vi "DoHandshake.vi"(6 "Additional Return headers (none)":T1[](array[typedef]), 8 "error in (no error)":errorcluster, 9 "timeout ms (5000)":i32=5000, 10 "Supported Protocols (any)":string[](array[string]), 11 "WebSocket Connection in":refnum<k5>) -> (0 "error out":errorcluster, 1 "Request URI":string, 2 "Headers Out":variant, 3 "WebSocket Connection out":refnum<k5>)   [LabVIEW 2013, in "WebSockets.lvlib"]
doc: "Performs the WebSockets HTTP handshaking on the new TCP connection. The client sends HTTP headers and the server must reply with a correctly formed HTTP response. The VI handles an incoming WS-Protocol and will return it in the response headers if it matches the supported protocols input. Additional HTTP headers can also be returned."
uses:
  WebSockets.lvlib
  Headers.ctl
panel:
  out "HTTP Headers":string
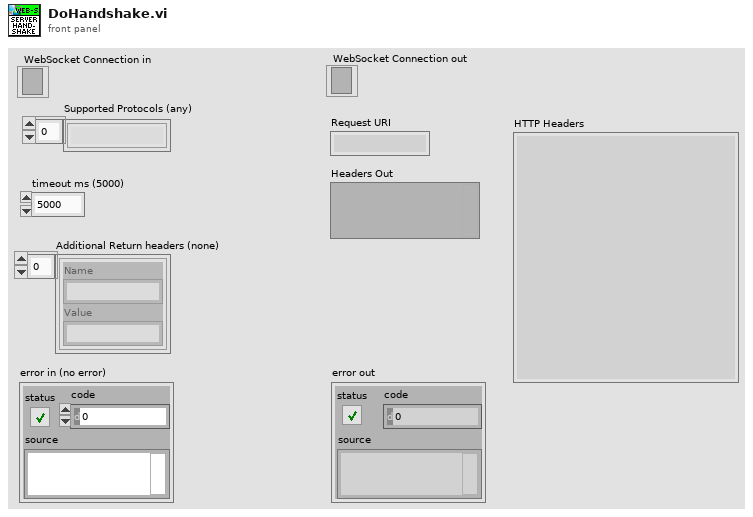
[diagram p1: front panel]
types:
  T1 = typedef "WebSockets.lvlib/Headers.ctl" = cluster{"Name":string, "Value":string}
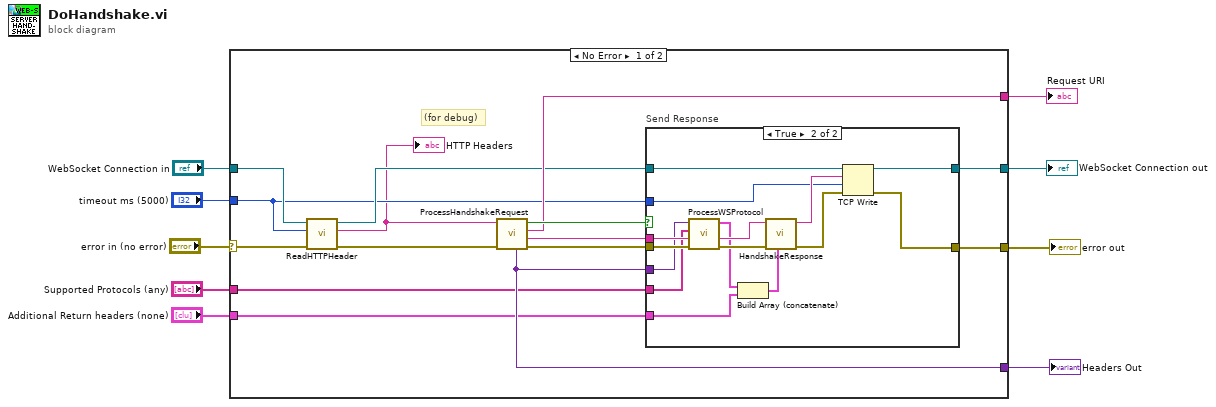
[diagram p0: block diagram]
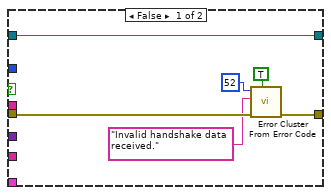
[diagram p2: hidden frame]
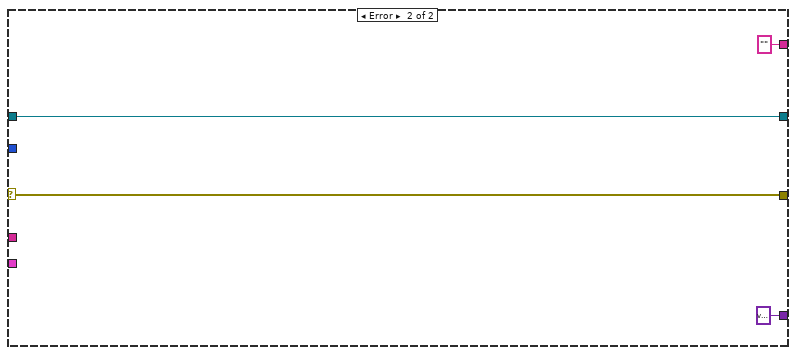
[diagram p3: hidden frame]
diagram:
  n1 = case shown="No Error" "error in (no error)" {
    selector: "error in (no error)" -> [w17 w48]
    tunnel: [w24 w47] -> w9
    tunnel: "WebSocket Connection in" -> [w18 w47]
    tunnel: [w20 w48] -> w6
    tunnel: "timeout ms (5000)" -> [w14 _]
    tunnel: [w12 variant ("Headers Out")] -> w4
    tunnel: [w19 "" ("Path")] -> w3
    tunnel: "Supported Protocols (any)" -> [w11 _]
    tunnel: "Additional Return headers (none)" -> [w10 _]
    frame No Error {
      # "(for debug)"
      n2 = call "ReadHTTPHeader.vi"("error in (no error)"=w17, "timeout ms (25000)"=w14, "WebSocket Connection in"=w18) -> ("error out"=w16:errorcluster, "HTTP Header"=w13:string, "WebSocket Connection out"=w15:refnum<k5>)  [unwired: 6 in]
      "HTTP Headers" <- w13
      n3 = call "ProcessHandshakeRequest.vi"("error in (no error)"=w16, "HTTP Headers"=w13) -> ("error out"=w21:errorcluster, "Sec-WebSocket-Key"=w23:string, "Path"=w19:string, "Is Websocket Request?"=w22:bool, "Headers Out"=w12:variant)  [unwired: 4 in, 1 out]
      n4 = case "Send Response" shown="True" w22 {
        tunnel: w23 -> [_ w44]
        tunnel: w15 -> [w30 w42]
        tunnel: [w30 w41] -> w24
        tunnel: w21 -> [w28 w37]
        tunnel: [w29 w39] -> w20
        tunnel: w14 -> [_ w38]
        tunnel: w12 -> [_ w35]
        tunnel: w11 -> [_ w33]
        tunnel: w10 -> [_ w31]
        frame False {
          n5 = call <vilib>:"Error Cluster From Error Code.vi"("show call chain? (False)"=TRUE, "error in (no error)"=w28, "error message (\"\")"="Invalid handshake data received." ("error message (\"\")"), "error code (0)"=52) -> ("error out"=w29:errorcluster)  [unwired: 5 in]
        }
        frame True {
          n6 = call "ProcessWSProtocol.vi"("error in (no error)"=w37, "Supported Protocols (any)"=w33, "Headers In"=w35) -> ("error out"=w36:errorcluster, "Protocol Header"=w34:T1[])  [unwired: 7 in]
          n7 = Build Array (concatenate)(w34, w31) -> (w32:T1[])
          n8 = call "HandshakeResponse.vi"("additional headers (none)"=w32, "error in (no error)"=w36, "Sec-WebSocket-Key"=w44) -> ("error out"=w40:errorcluster, "Response Headers"=w43:string)  [unwired: 7 in]
          n9 = TCP Write(connection ID=w42, data in=w43, error in (no error)=w40, 9:w38) -> (connection ID out=w41:refnum<k5>, error out=w39:errorcluster)  [unwired: 1 out]
        }
      }
    }
    frame Error {
    }
  }
  "WebSocket Connection out" <- w9
  "error out" <- w6
  "Headers Out" <- w4
  "Request URI" <- w3
